vi "Register.Initialize.vi"(8 "error in (no error)":errorcluster, 10 "Register":T3={"Name"="", "Data Type"=enum."<Null>", "Default Value"=variant(dbl 0.0)} {"Data Type" format="%.0x"}, 11 "FPGA Ref":refnum<k20>) -> (0 "error out":errorcluster, 2 "Register out":T1 {"Data Type" format="%.0x"}, 3 "FPGA Ref out":refnum<k20>)   [LabVIEW 2019, in "Fuel Injector Analysis Addon Engine.lvlib"]
uses:
  Fuel Injector Analysis Addon Engine.lvlib
  <vilib>/NI/LVFPGA Adv Session Resources/OpenByName.xnode
  Addon Shared/Types/FPGA Data Types.ctl
  Addon Shared/Fuel Injector Analysis Addon Shared.lvlib
  Types/FPGA Refs.ctl
  <vilib>/NI/LVFPGA Adv Session Resources/OpenByNameSubVI.vi
  <vilib>/NI/LVFPGA Adv Session Resources/LVFPGAAdvSessionResources.lvlib
  Addon Shared/Types/Register.Info.ctl
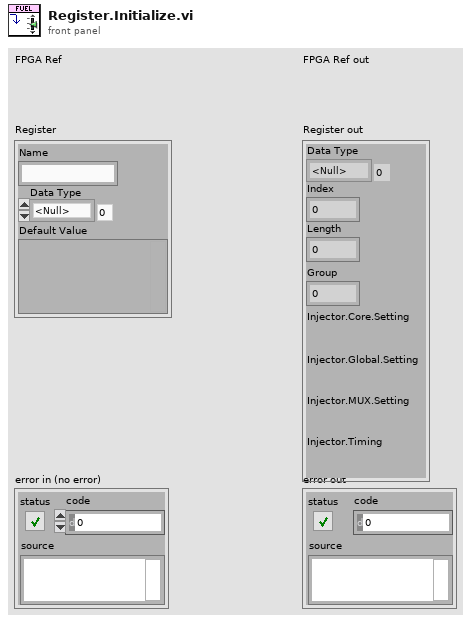
[diagram p1: front panel]
types:
  T1 = typedef "Fuel Injector Analysis Addon Engine.lvlib/FPGA Refs.ctl" = cluster{"Data Type":T2, "Index":i32, "Length":i32, "Group":i32, "Injector.Core.Setting":refnum<k20>, "Injector.Global.Setting":refnum<k20>, "Injector.MUX.Setting":refnum<k20>, "Injector.Timing":refnum<k20>}
  T2 = typedef "Fuel Injector Analysis Addon Shared.lvlib/FPGA Data Types.ctl" = enum8{"<Null>", "Injector.Core.Setting", "Injector.Global.Setting", "Injector.Mux.Setting", "Injector.Timing"}
  T3 = typedef "Fuel Injector Analysis Addon Shared.lvlib/Register.Info.ctl" = cluster{"Name":string, "Data Type":T2, "Default Value":variant}
  T4 = cluster{"Name":string, "Depth":u32, "Write? (Deprecated:Use Implementation)":bool, "Physical Channel":u32, "Base Address":u32, "Data Width":u32, "Data Type":enum32{"Boolean", "I8", "I16", "I32", "I64", "U8", "U16", "U32", "U64", "FXP", "CustomControl", "SGL"}, "FXP Properties":variant, "Write Window Address":u32, "Implementation":enum16{"niFpgaTargetToHost", "niFpgaHostToTarget", "niFpgaPeerToPeerWriter", "niFpgaPeerToPeerReader", "niCoreTargetToHost", "niCoreHostToTarget"}, "Control Set":u32}[]
  T5 = cluster{"Name":string, "type":variant, "indicator?":bool}[]
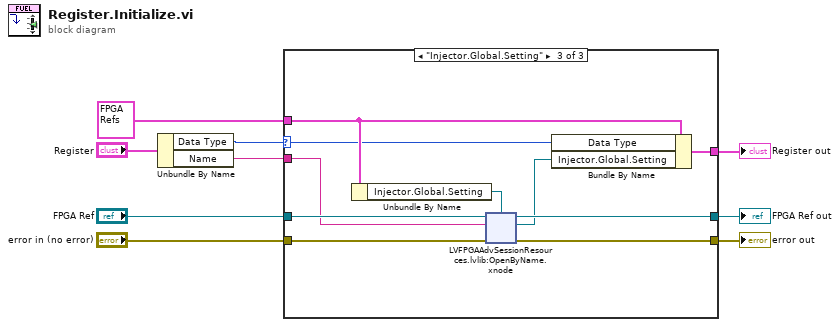
[diagram p0: block diagram]
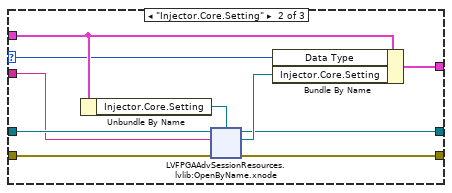
[diagram p3: hidden frame]
diagram:
  n1 = Unbundle By Name("Register") -> ("Data Type"=w2:T2, "Name"=w1:string)
  n2 = case shown="\"Injector.Global.Setting\"" w2 {
    selector: w2 -> [_ w18 w40]
    tunnel: [w11 w14 w45] -> w9
    tunnel: [w12 w13 w37] -> w8
    tunnel: "FPGA Ref" -> [w11 w22 w44]
    tunnel: "error in (no error)" -> [w12 w16 w38]
    tunnel: [w10 w21 w43] -> w4
    tunnel: T1 {"Data Type"=enum."<Null>", "Index"=0, "Length"=0, "Group"=0, "Injector.Core.Setting"=refnum, "Injector.Global.Setting"=refnum, "Injector.MUX.Setting"=refnum, "Injector.Timing"=refnum} ("Register") -> [w10 w20 w42]
    tunnel: w1 -> [_ w17 w39]
    frame "<Null>", Default {
    }
    frame "Injector.Core.Setting" {
      n3 = Unbundle By Name(w20) -> ("Injector.Core.Setting"=w19:refnum<k20>)
      n4 = xnode "LVFPGAAdvSessionResources.lvlib:OpenByName.xnode"("FPGA VI Reference in"=w22, "Resource name in"=w17, "Single resource reference type in"=w19, "Error in"=w16) -> ("Single resource reference out"=w15:refnum<k20>, "Error out"=w13:errorcluster, "FPGA VI Reference out"=w14:refnum<k20>)
      n5 = Bundle By Name(cluster=w20, "Data Type"=w18, "Injector.Core.Setting"=w15) -> (w21:T1)
    }
    frame "Injector.Global.Setting" {
      n6 = Unbundle By Name(w42) -> ("Injector.Global.Setting"=w41:refnum<k20>)
      n7 = xnode "LVFPGAAdvSessionResources.lvlib:OpenByName.xnode"("FPGA VI Reference in"=w44, "Resource name in"=w39, "Single resource reference type in"=w41, "Error in"=w38) -> ("Single resource reference out"=w36:refnum<k20>, "Error out"=w37:errorcluster, "FPGA VI Reference out"=w45:refnum<k20>)
      n8 = Bundle By Name(cluster=w42, "Data Type"=w40, "Injector.Global.Setting"=w36) -> (w43:T1)
    }
  }
  "FPGA Ref out" <- w9
  "error out" <- w8
  "Register out" <- w4
